vi "global_raw.vi"() -> ()   [LabVIEW 2021]
panel:
  out "Datos Leídos Luz":string[](array[string])
  out "Datos Leídos T y P":string[](array[string])
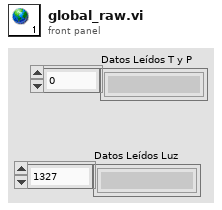
[diagram p1: front panel]
diagram:
